vi "Climber.vi"   [LabVIEW 2012]
uses:
  <vilib>/Rock Robotics/WPI/Solenoid/WPI_SolenoidValue.ctl
  <vilib>/Rock Robotics/WPI/Joystick/WPI_JoystickGetSetRefNum.vi
  <vilib>/Rock Robotics/WPI/Solenoid/WPI_SolenoidSetEnum.vi
types:
  T1 = typedef "WPI_JoystickDevRef.ctl" = cluster{"Device":T2}
  T2 = typedef "WPI_JoystickDeviceEnum.ctl" = enum16{"USB 1", "USB 2", "USB 3", "USB 4", "Kinect 1", "Kinect 2"}
  T3 = typedef "WPI_JoystickButtonState.ctl" = cluster{"Button 1":bool, "Button 2":bool, "Button 3":bool, "Button 4":bool, "Button 5":bool, "Button 6":bool, "Button 7":bool, "Button 8":bool, "Button 9":bool, "Button 10":bool, "Button 11":bool, "Button 12":bool}
  T4 = cluster{"axis 1 (x)":dbl, "axis 2 (y)":dbl, "axis 3 (throttle)":dbl, "axis 4":dbl, "axis 5":dbl, "axis 6":dbl}
  T5 = typedef "WPI_SolenoidValue.ctl" = enum16{"Off", "On", "Forward", "Reverse"}
  T6 = typedef "WPI_SolenoidDevRef.ctl" = cluster{"DevStatus":errorcluster, "Solenoid Module":T7, "Forward Solenoid Channel":T8, "Reverse Solenoid Channel":T8}
  T7 = typedef "FPGA_TypedefSolenoidModule.ctl" = enum16{"Solenoid Module 1", "Solenoid Module 2"}
  T8 = typedef "WPI_SolenoidChannel.ctl" = enum8{"Solenoid 1", "Solenoid 2", "Solenoid 3", "Solenoid 4", "Solenoid 5", "Solenoid 6", "Solenoid 7", "Solenoid 8", "Invalid"}
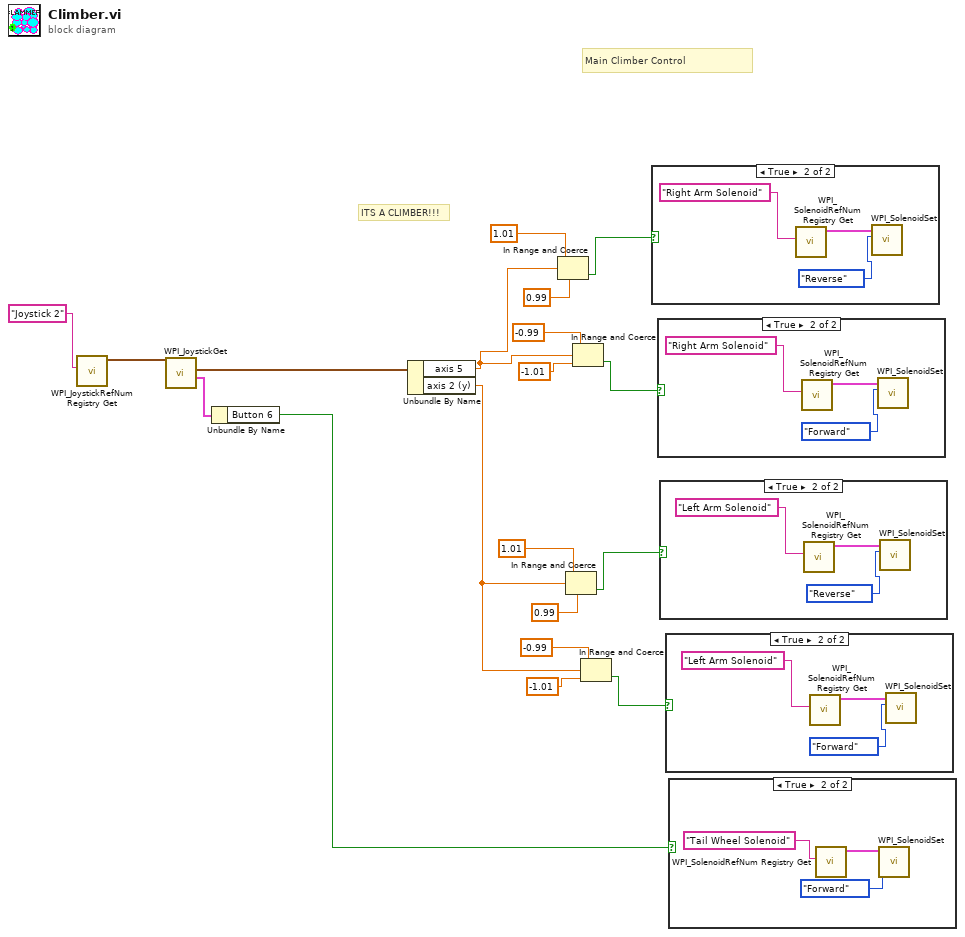
[diagram p0: block diagram]
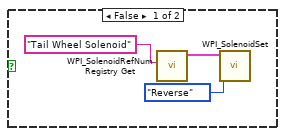
[diagram p2: hidden frame]
diagram:
  # "ITS A CLIMBER!!!"
  # "Main Climber Control"
  n1 = call <vilib>:"WPI_JoystickRefNum Registry Get.vi"("refnum name"="Joystick 2") -> ("JoystickDevRef"=w18:T1)  [unwired: 9 in, 1 out]
  n2 = call <vilib>:"WPI_JoystickGet.vi"("JoystickDevRef"=w18) -> ("Buttons"=w2:T3, "Axes"=w17:T4)  [unwired: 4 in, 1 out]
  n3 = Unbundle By Name(w2) -> ("Button 6"=w1:bool)
  n4 = Unbundle By Name(w17) -> ("axis 5"=w11:dbl, "axis 2 (y)"=w3:dbl)
  n5 = In Range and Coerce(upper limit=1.01, x=w11, lower limit=0.99) -> (In Range?=w14:bool)  [unwired: 1 out]
  n6 = In Range and Coerce(upper limit=1.01, x=w3, lower limit=0.99) -> (In Range?=w7:bool)  [unwired: 1 out]
  n7 = In Range and Coerce(upper limit=-0.99, x=w11, lower limit=-1.01) -> (In Range?=w10:bool)  [unwired: 1 out]
  n8 = In Range and Coerce(upper limit=-0.99, x=w3, lower limit=-1.01) -> (In Range?=w4:bool)  [unwired: 1 out]
  n9 = case shown="True" w14 {
    frame False {
    }
    frame True {
      n10 = call <vilib>:"WPI_SolenoidRefNum Registry Get.vi"("refnum name"="Right Arm Solenoid") -> ("SolenoidDevRef"=w21:T6)  [unwired: 9 in, 1 out]
      n11 = call-poly <vilib>:"WPI_SolenoidSet.vi"("Value"=WPI_SolenoidValue."Reverse", "SolenoidDevRef"=w21) -> ()  [unwired: 8 in, 2 out]
    }
  }
  n12 = case shown="True" w10 {
    frame False {
    }
    frame True {
      n13 = call <vilib>:"WPI_SolenoidRefNum Registry Get.vi"("refnum name"="Right Arm Solenoid") -> ("SolenoidDevRef"=w24:T6)  [unwired: 9 in, 1 out]
      n14 = call-poly <vilib>:"WPI_SolenoidSet.vi"("Value"=WPI_SolenoidValue."Forward", "SolenoidDevRef"=w24) -> ()  [unwired: 8 in, 2 out]
    }
  }
  n15 = case shown="True" w7 {
    frame False {
    }
    frame True {
      n16 = call <vilib>:"WPI_SolenoidRefNum Registry Get.vi"("refnum name"="Left Arm Solenoid") -> ("SolenoidDevRef"=w27:T6)  [unwired: 9 in, 1 out]
      n17 = call-poly <vilib>:"WPI_SolenoidSet.vi"("Value"=WPI_SolenoidValue."Reverse", "SolenoidDevRef"=w27) -> ()  [unwired: 8 in, 2 out]
    }
  }
  n18 = case shown="True" w4 {
    frame False {
    }
    frame True {
      n19 = call <vilib>:"WPI_SolenoidRefNum Registry Get.vi"("refnum name"="Left Arm Solenoid") -> ("SolenoidDevRef"=w30:T6)  [unwired: 9 in, 1 out]
      n20 = call-poly <vilib>:"WPI_SolenoidSet.vi"("Value"=WPI_SolenoidValue."Forward", "SolenoidDevRef"=w30) -> ()  [unwired: 8 in, 2 out]
    }
  }
  n21 = case shown="True" w1 {
    frame False {
      n22 = call <vilib>:"WPI_SolenoidRefNum Registry Get.vi"("refnum name"="Tail Wheel Solenoid") -> ("SolenoidDevRef"=w33:T6)  [unwired: 9 in, 1 out]
      n23 = call-poly <vilib>:"WPI_SolenoidSet.vi"("Value"=WPI_SolenoidValue."Reverse", "SolenoidDevRef"=w33) -> ()  [unwired: 8 in, 2 out]
    }
    frame True {
      n24 = call <vilib>:"WPI_SolenoidRefNum Registry Get.vi"("refnum name"="Tail Wheel Solenoid") -> ("SolenoidDevRef"=w36:T6)  [unwired: 9 in, 1 out]
      n25 = call-poly <vilib>:"WPI_SolenoidSet.vi"("Value"=WPI_SolenoidValue."Forward", "SolenoidDevRef"=w36) -> ()  [unwired: 8 in, 2 out]
    }
  }
